vi "CleanUpNode.vi"(8 "error in":errorcluster, 10 "Parameters":variant, 11 "module editor node in":refnum<class "module editor node.lvclass">) -> (0 "error out":errorcluster, 3 "module editor node out":refnum<class "module editor node.lvclass">)   [LabVIEW 2013, in "PL Framework Configuration Tool.lvlib" / "module editor node.lvclass"]
doc: "This VI will clean any reference handled internally in the node"
uses:
  module editor node.lvclass
  <vilib>/NI/Configuration Framework/serializable configuration/NISE_CEF_serializable configuration.lvclass/NISE_CEF_serializable configuration.ctl
  <vilib>/NI/Configuration Framework/serializable configuration/NISE_CEF_serializable configuration.lvclass
  <vilib>/NI/Module Execution Interface/Engine Configuration/engine configuration.lvclass
  Read Module Configuration.vi
  Engine Parent/read engine configuration.vi
  Engine Parent/write engine configuration.vi
  <vilib>/NI/Tag Bus Module Framework/module configuration/TBM module configuration.lvclass
  Engine Parent/Engine Parent Editor Node.lvclass
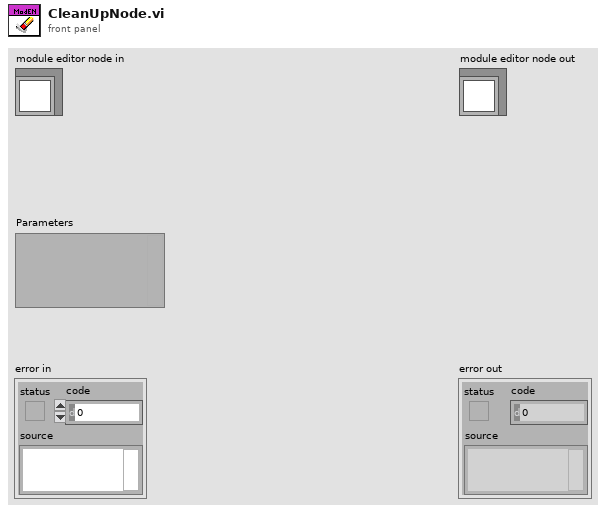
[diagram p1: front panel]
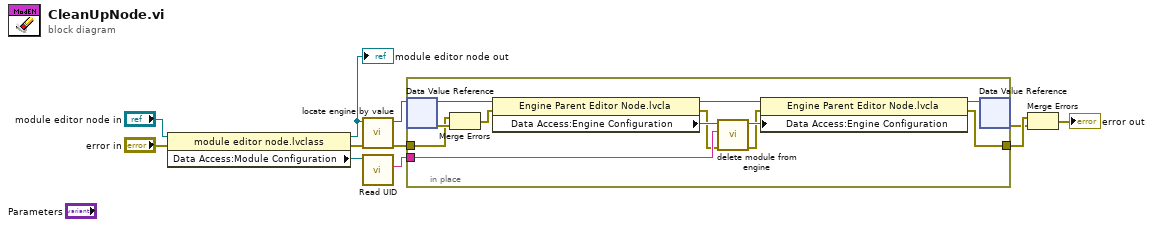
[diagram p0: block diagram]
diagram:
  n1 = property class="module editor node.lvclass"(reference="module editor node in", error in="error in") -> (reference out=w8:refnum<class "module editor node.lvclass">, error out=w10:errorcluster, "Data Access:Module Configuration"=w7:refnum<class "TBM module configuration.lvclass">)
  "module editor node out" <- w8
  n2 = call "locate engine by value.vi"("error in"=w10, "Node"=w8) -> ("error out"=w4:errorcluster, "engine"=w5:refnum<data-value>)  [unwired: 8 in]
  n3 = call <vilib>:"Read UID.vi"("configuration in"=w7) -> ("instance id"=w6:string)  [unwired: 8 in, 2 out]
  n4 = in-place {
    in-place-border: w6 -> [w20]
    in-place-border: w4 -> [w18]
    in-place-border: [w12] -> w3
    n5 = in-place-dvr #1(w5) -> (w16:refnum<class "Engine Parent Editor Node.lvclass">, w19:errorcluster)
    n6 = Merge Errors(w18, w19) -> (w17:errorcluster)
    n7 = property class="Engine Parent Editor Node.lvcla"(reference=w16, error in=w17) -> (reference out=w23:refnum<class "Engine Parent Editor Node.lvclass">, error out=w14:errorcluster, "Data Access:Engine Configuration"=w22:refnum<class "engine configuration.lvclass">)
    n8 = call-dynamic "delete module from engine.vi"("error in"=w14, "module ID"=w20, "engine configuration in"=w22) -> ("error out"=w13:errorcluster, "engine configuration out"=w21:refnum<class "engine configuration.lvclass">)  [unwired: 7 in]
    n9 = property class="Engine Parent Editor Node.lvcla"(reference=w23, error in=w13, "Data Access:Engine Configuration"=w21) -> (reference out=w15:refnum<class "Engine Parent Editor Node.lvclass">, error out=w12:errorcluster)
    n10 = in-place-dvr #1(w15) -> (w2:errorcluster)  [unwired: 1 out]
  }
  n11 = Merge Errors(w3, w2) -> (→"error out":errorcluster)
